vi "MinMaxArray.vi"() -> ()   [LabVIEW 2014]
panel:
  out "sorted array":dbl[](array[numeric])
  out "min value":dbl
  out "max value":dbl
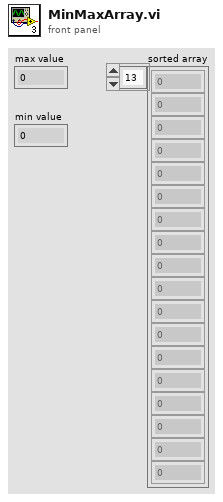
[diagram p1: front panel]
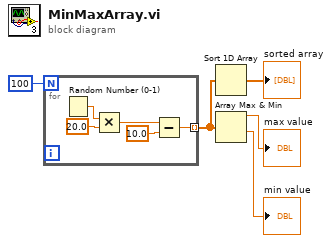
[diagram p0: block diagram]
diagram:
  n1 = for {
    N: 100 -> [_]
    tunnel: [w6] -> w2 mode=indexing
    n2 = Random Number (0-1)() -> (number: 0 to 1=w10:dbl)
    n3 = Multiply(x=w10, y=20.0) -> (x*y=w8:dbl)
    n4 = Subtract(x=w8, y=10.0) -> (x-y=w6:dbl)
  }
  n5 = Sort 1D Array(array=w2) -> (sorted array=→"sorted array":dbl[])
  n6 = Array Max & Min(array=w2) -> (max value=→"max value":dbl, min value=→"min value":dbl)  [unwired: 2 out]
